vi "FIR Windowed Filter Design.vi"() -> ()   [LabVIEW 2023]
doc: "This example shows the Transfer Function of an FIR windowed filter given the filter type. The parameters are different for each filter type and may be changed to investigate their effect on the response."
uses:
  <vilib>/Utility/error.llb/DialogType.ctl
  <vilib>/Analysis/3filter.llb/FIR Windowed Filter (DBL).vi
  <vilib>/Analysis/NI_AALPro.lvlib
  <vilib>/Analysis/NI_AALBase.lvlib
  <vilib>/measure/NI_MAPro.lvlib
panel:
  out "Error Message":string
  out "Phase Response":cluster{dbl, dbl, dbl[]}(graph)
  out "Magnitude Response":cluster{dbl, dbl, dbl[]}(graph)
  in  "window":u32(ring) items=["Rectangle"=0, "Hanning"=1, "Hamming"=2, "Blackman-Harris"=3, "Exact Blackman"=4, "Blackman"=5, "Flat Top"=6, "4 Term B-Harris "=7, "7 Term B-Harris"=8, "Low Sidelobe"=9, "Blackman Nuttall"=11, "Triangle"=30, "Bartlett-Hanning"=31, "Bohman"=32, "Parzen"=33, "Welch"=34, "Kaiser"=60, "Dolph-Chebyshev"=61, "Gaussian"=62]
  in  "filter type":T1(ring)
  in  "high cutoff freq: fh":dbl=350.0 format="%#.6g"
  in  "low cutoff freq: fl":dbl=150.0 format="%#.6g"
  in  "sampling frequency: fs":dbl=1000.0 format="%#.6g"
  in  "Stop":bool
  in  "taps":i32=33
  # "Overview: Demonstrates the design options for windowed FIR filter design.\nRequirements: LabVIEW Full Development System\nInstructions:\n1. Run the VI.\n2. Manipulate the parameters and observe the results in the Magnitude Response and Phase Response graphs.\n3. Click Stop to stop the VI."
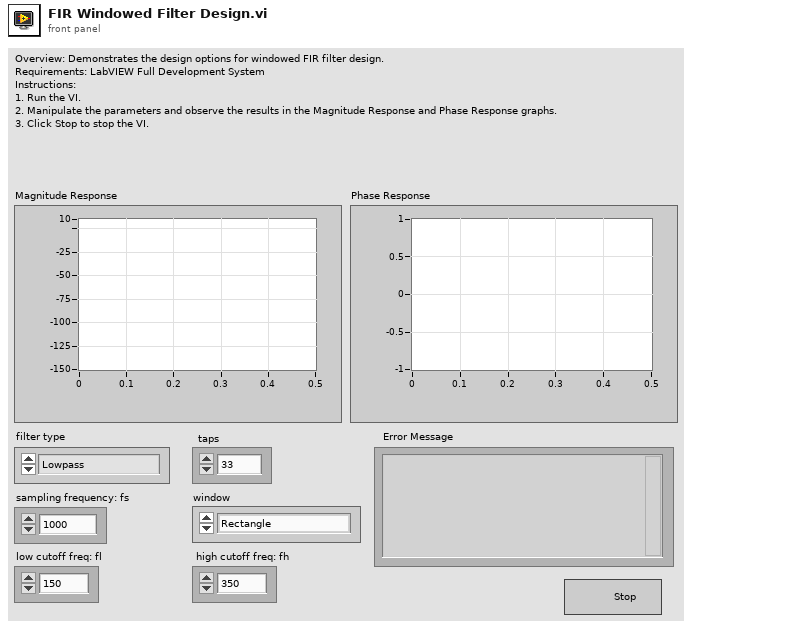
[diagram p1: front panel]
types:
  T1 = enum32{"Lowpass", "Highpass", "Bandpass", "Bandstop"}
  T2 = enum32{"Vrms", "Vpk", "Vrms^2", "Vpk^2", "Vrms/rtHz", "Vpk/rtHz", "Vrms^2/Hz", "Vpk^2/Hz"}
  T3 = enum16{"Power (Vrms^2)", "Amplitude (Vrms)", "Gain (amplitude ratio)"}
  T4 = typedef "DialogType.ctl" = u16
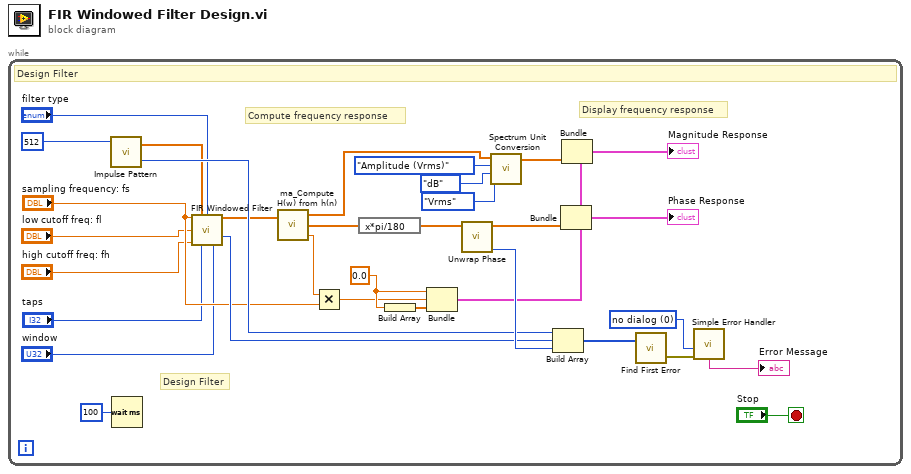
[diagram p0: block diagram]
diagram:
  n1 = while {
    stop <- "Stop" stop-if-true
    w2 = T4 0 items=["no dialog", "OK message", "continue or stop message", "OK message + warnings", "continue/stop + warnings"] ("type of dialog (OK msg:1)")
    w28 = 0.0
    # "Display frequency response"
    # "Compute frequency response"
    # "Design Filter"
    # "Design Filter"
    n2 = call <vilib>:"Impulse Pattern.vi"("samples"=512) -> ("error"=w31:i32, "Impulse Pattern"=w22:dbl[])  [unwired: 2 in]
    n3 = Wait (ms)(milliseconds to wait=u32 100) -> ()  [unwired: 1 out]
    n4 = call-poly <vilib>:"FIR Windowed Filter.vi"("sampling freq: fs"="sampling frequency: fs", "X"=w22, "filter type"="filter type", "low cutoff freq: fl"="low cutoff freq: fl", "high cutoff freq: fh"="high cutoff freq: fh", "taps"="taps", "window"="window") -> ("Filtered X"=w5:dbl[], "error"=w32:i32)  [unwired: 7 in]
    n5 = call <vilib>:"ma_Compute H(w) from h(n).vi"("h"=w5) -> ("Mag H(w)"=w11:dbl[], "Phase H(w)"=w9:dbl[], "df"=w7:dbl)  [unwired: 1 in]
    n6 = Multiply(x=w7, y="sampling frequency: fs") -> (x*y=w27:dbl)
    n7 = expression code="x*pi/180"(w9) -> (w8:dbl[])
    n8 = Build Array ("array")(w28) -> (w29:dbl[])
    n9 = Bundle(w28, w27, w29) -> (w24:cluster{dbl, dbl, dbl[]})  [unwired: 1 in]
    n10 = call <vilib>:"Unwrap Phase.vi"("Phase"=w8) -> ("error"=w33:i32, "Unwrapped Phase"=w25:dbl[])  [unwired: 9 in]
    n11 = call <vilib>:"Spectrum Unit Conversion.vi"("display unit"=T2."Vrms", "log/linear"=enum16{"Linear", "dB", "dBm"}."dB", "spectrum type"=T3."Amplitude (Vrms)", "Spectrum in"=w11) -> ("Spectrum out"=w10:dbl[])  [unwired: 6 in, 1 out]
    n12 = Build Array(w31, w32, w33) -> (w4:i32[])
    n13 = Bundle(cluster=w24, w25) -> (→"Phase Response":cluster{dbl, dbl, dbl[]})  [unwired: 2 in]
    n14 = Bundle(cluster=w24, w10) -> (→"Magnitude Response":cluster{dbl, dbl, dbl[]})  [unwired: 2 in]
    n15 = call <vilib>:"Find First Error.vi"("error codes"=w4) -> ("error out"=w1:errorcluster)  [unwired: 3 in, 1 out]
    n16 = call <vilib>:"Simple Error Handler.vi"("type of dialog (OK msg:1)"=w2, "error in (no error)"=w1) -> ("message"=→"Error Message":string)  [unwired: 3 in, 4 out]
  }
